vi "testBenchmarkSystemDefinition.vi"(8 "error in (no error)":errorcluster, 11 "TestCase in":refnum<class "VeriStandTestCaseTests.lvclass">) -> (0 "error out":errorcluster, 3 "TestCase out":refnum<class "VeriStandTestCaseTests.lvclass">)   [LabVIEW 2015, in "VeriStandTestCaseTests.lvclass"]
uses:
  VeriStandTestCaseTests.lvclass
  VeriStandTestCase.lvclass
  <vilib>/addons/_JKI Toolkits/VI Tester/TestCase.llb/TestCase.lvclass
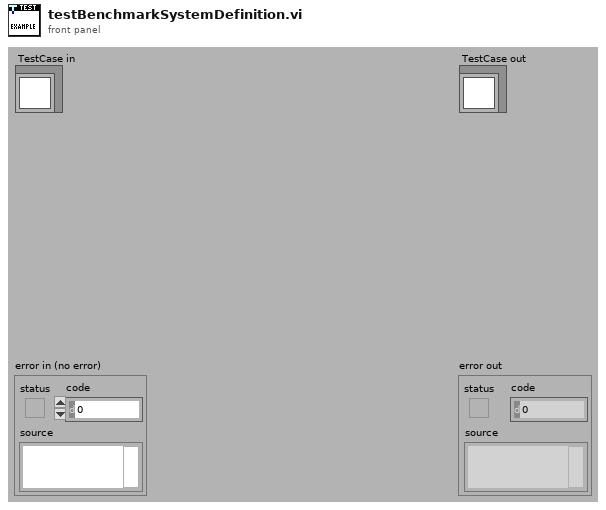
[diagram p1: front panel]
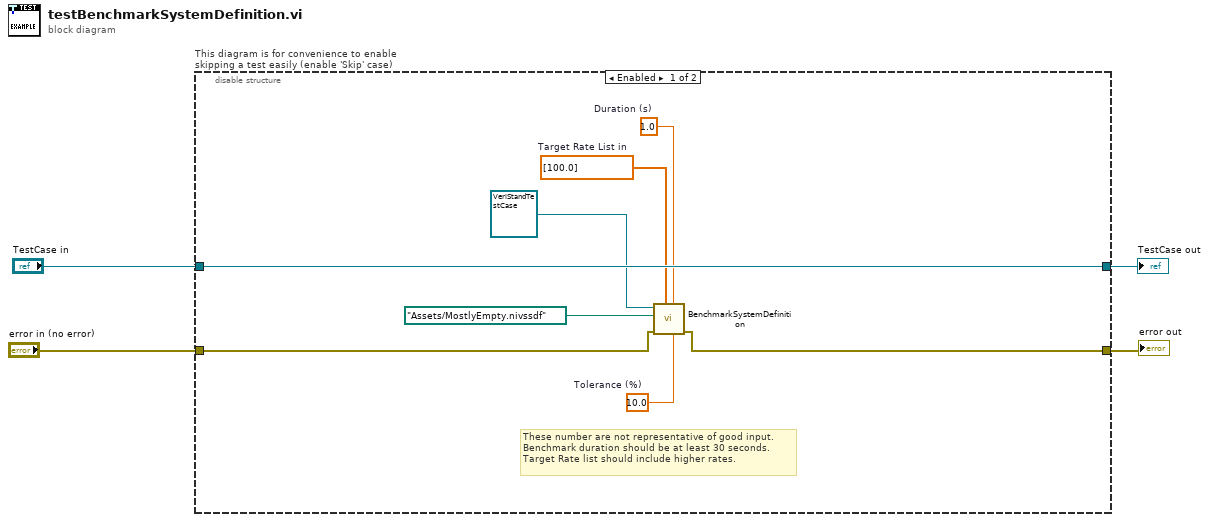
[diagram p0: block diagram]
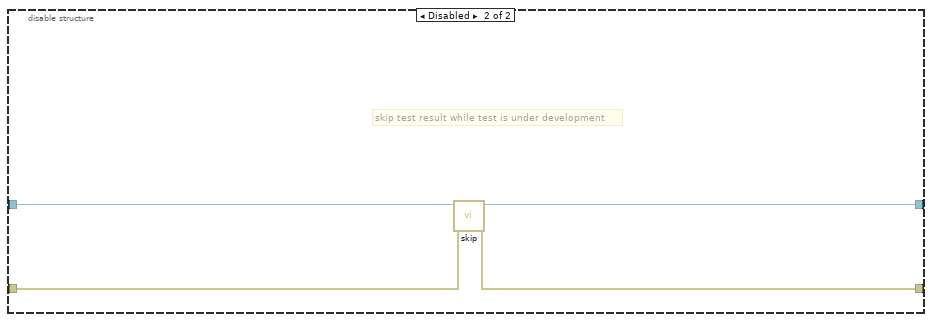
[diagram p2: hidden frame]
diagram:
  n1 = disable-structure "This diagram is for convenience to enable skipping a test easily (enable 'Skip' case)" shown="Enabled" {
    disable-tunnel: "TestCase in" -> [w12 w16]
    disable-tunnel: [w12 w14] -> w1
    disable-tunnel: [w10 w15] -> w3
    disable-tunnel: "error in (no error)" -> [w11 w13]
    frame Enabled {
      w5 = 10.0  # Tolerance (%)
      w6 = 1.0  # Duration (s)
      w7 = dbl[] [100.0]  # Target Rate List in
      # "These number are not representative of good input.\nBenchmark duration should be at least 30 seconds.\nTarget Rate list should include higher rates."
      n2 = call-dynamic "BenchmarkSystemDefinition.vi"("Tolerance (%)"=w5, "Duration (s)"=w6, "Target Rate List in"=w7, "error in (no error)"=w11, "System Definition File"=path "Assets/MostlyEmpty.nivssdf", "VeriStandTestCase in"=refnum<class "VeriStandTestCase.lvclass"> refnum ("VeriStand Test Case in")) -> ("error out"=w10:errorcluster)  [unwired: 4 in, 1 out]
    }
    frame Disabled {
      # "skip test result while test is under development"
      n3 = call <vilib>:"skip.vi"("error in (no error)"=w13, "TestCase in"=w16) -> ("error out"=w15:errorcluster, "TestCase out"=w14:refnum<class "VeriStandTestCaseTests.lvclass">)  [unwired: 8 in]
    }
  }
  "error out" <- w3
  "TestCase out" <- w1
